vi "queueing files.vi"() -> ()   [LabVIEW 2014]
uses:
  <vilib>/Utility/file.llb/Write To Spreadsheet File (string).vi
  <vilib>/Utility/file.llb/Write To Spreadsheet File (DBL).vi
  <vilib>/Utility/file.llb/Read From Spreadsheet File (string).vi
panel:
  out "appended array 2":string[][](array[string])
  in  "Stop Button":bool
  out "appended array":dbl[][](array[numeric])
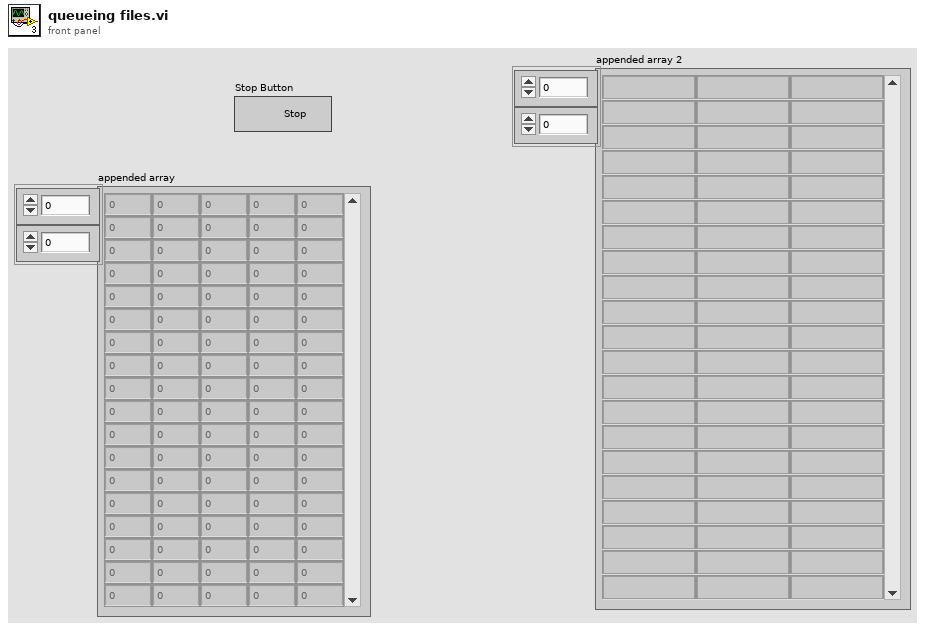
[diagram p1: front panel]
types:
  T1 = enum16{"open", "open or create", "create or replace", "create", "open (read only)"}
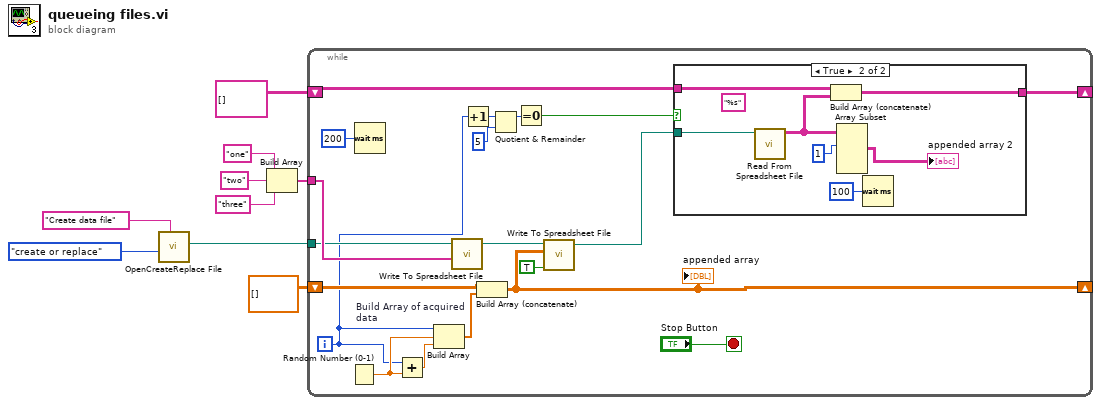
[diagram p0: block diagram]
diagram:
  n1 = call "OpenCreateReplace File.vi"("prompt"="Create data file", "function (open:0)"=T1."create or replace") -> ("new file path"=w2:path)  [unwired: 6 in, 3 out]
  n2 = Build Array("one" ("prompt"), "two" ("prompt"), "three" ("prompt")) -> (w3:string[])
  n3 = while {
    tunnel: w2 -> [w18]
    shift-right: [w25] -> _
    shift-left: dbl[][] [] -> [w26]
    tunnel: w3 -> [w19]
    shift-right: [w12] -> _
    shift-left: string[][] [] -> [w11]
    i -> [w15]
    stop <- "Stop Button" stop-if-true
    n4 = Random Number (0-1)() -> (number: 0 to 1=w23:dbl)
    n5 = Wait (ms)(milliseconds to wait=u32 200) -> ()  [unwired: 1 out]
    n6 = Add(x=w15, y=w23) -> (x+y=w22:dbl)
    n7 = Build Array "Build Array of acquired data"(w15, w23, w22) -> (w27:dbl[])
    n8 = call-poly <vilib>:"Write To Spreadsheet File.vi"("1D data"=w19, "file path (dialog if empty)"=w18) -> ("new file path (Not A Path if cancelled)"=w21:path)  [unwired: 6 in]
    n9 = Increment(x=w15) -> (x+1=w14:i32)
    n10 = Build Array (concatenate)(w26, w27) -> (w25:dbl[][])
    "appended array" <- w25
    n11 = Quotient & Remainder(x=w14, y=5) -> (x-y*floor(x/y)=w16:i32)  [unwired: 1 out]
    n12 = Equal To 0?(x=w16) -> (x = 0?=w13:bool)
    n13 = call-poly <vilib>:"Write To Spreadsheet File.vi"("append to file? (new file:F)"=TRUE, "2D data"=w25, "file path (dialog if empty)"=w21) -> ("new file path (Not A Path if cancelled)"=w10:path)  [unwired: 5 in]
    n14 = case shown="True" w13 {
      tunnel: w10 -> [_ w36]
      tunnel: [w29 w32] -> w12
      tunnel: w11 -> [w29 w31]
      frame False {
      }
      frame True {
        (unwired) "%s" ("format (%.3f)")
        n15 = call-poly <vilib>:"Read From Spreadsheet File.vi"("file path (dialog if empty)"=w36) -> ("all rows"=w33:string[][])  [unwired: 6 in, 4 out]
        n16 = Build Array (concatenate)(w31, w33) -> (w32:string[][])
        n17 = Array Subset(array=w33, index (row)=1 ("index")) -> (→"appended array 2":string[][])  [unwired: 3 in]
        n18 = Wait (ms)(milliseconds to wait=u32 100) -> ()  [unwired: 1 out]
      }
    }
  }
